vi "Plot_lift_off.vi"() -> ()   [LabVIEW 2018]
panel:
  in  "Raw/Pro":bool
  in  "Backdata":bool=TRUE caption="Scan"
  in  "Exit":bool
  in  "2D Array In":dbl[][](array[numeric])
  in  "Open":bool
  out "Hall sensors signal lf":dbl[][](graph)
  in  "Filter lf":bool=TRUE caption="Scan"
  in  "View Mode":bool caption="Scan"
  in  "Low cutoff freq: fl":dbl
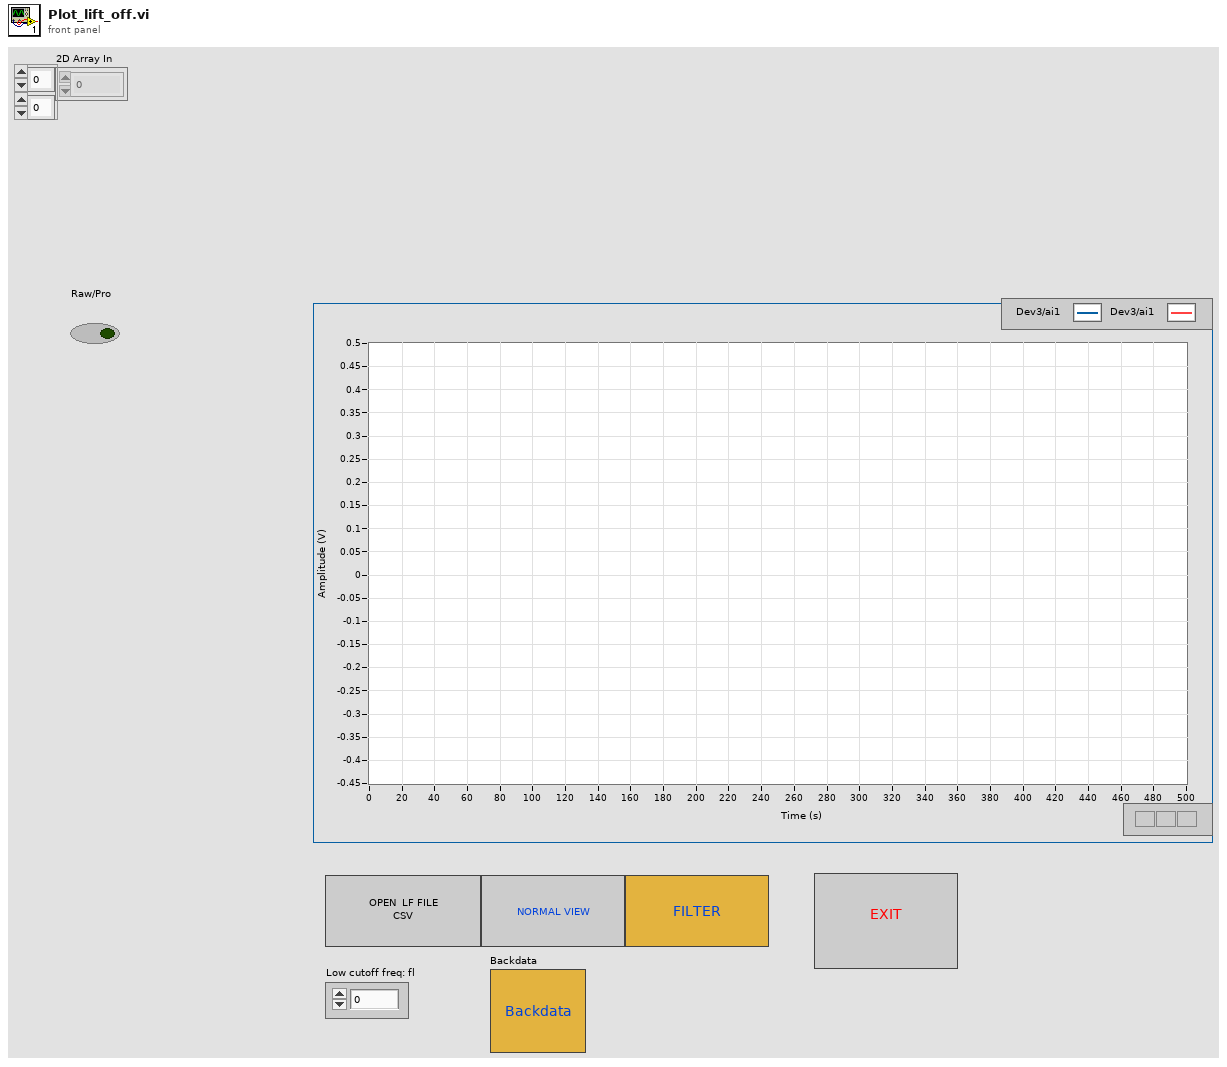
[diagram p1: front panel]
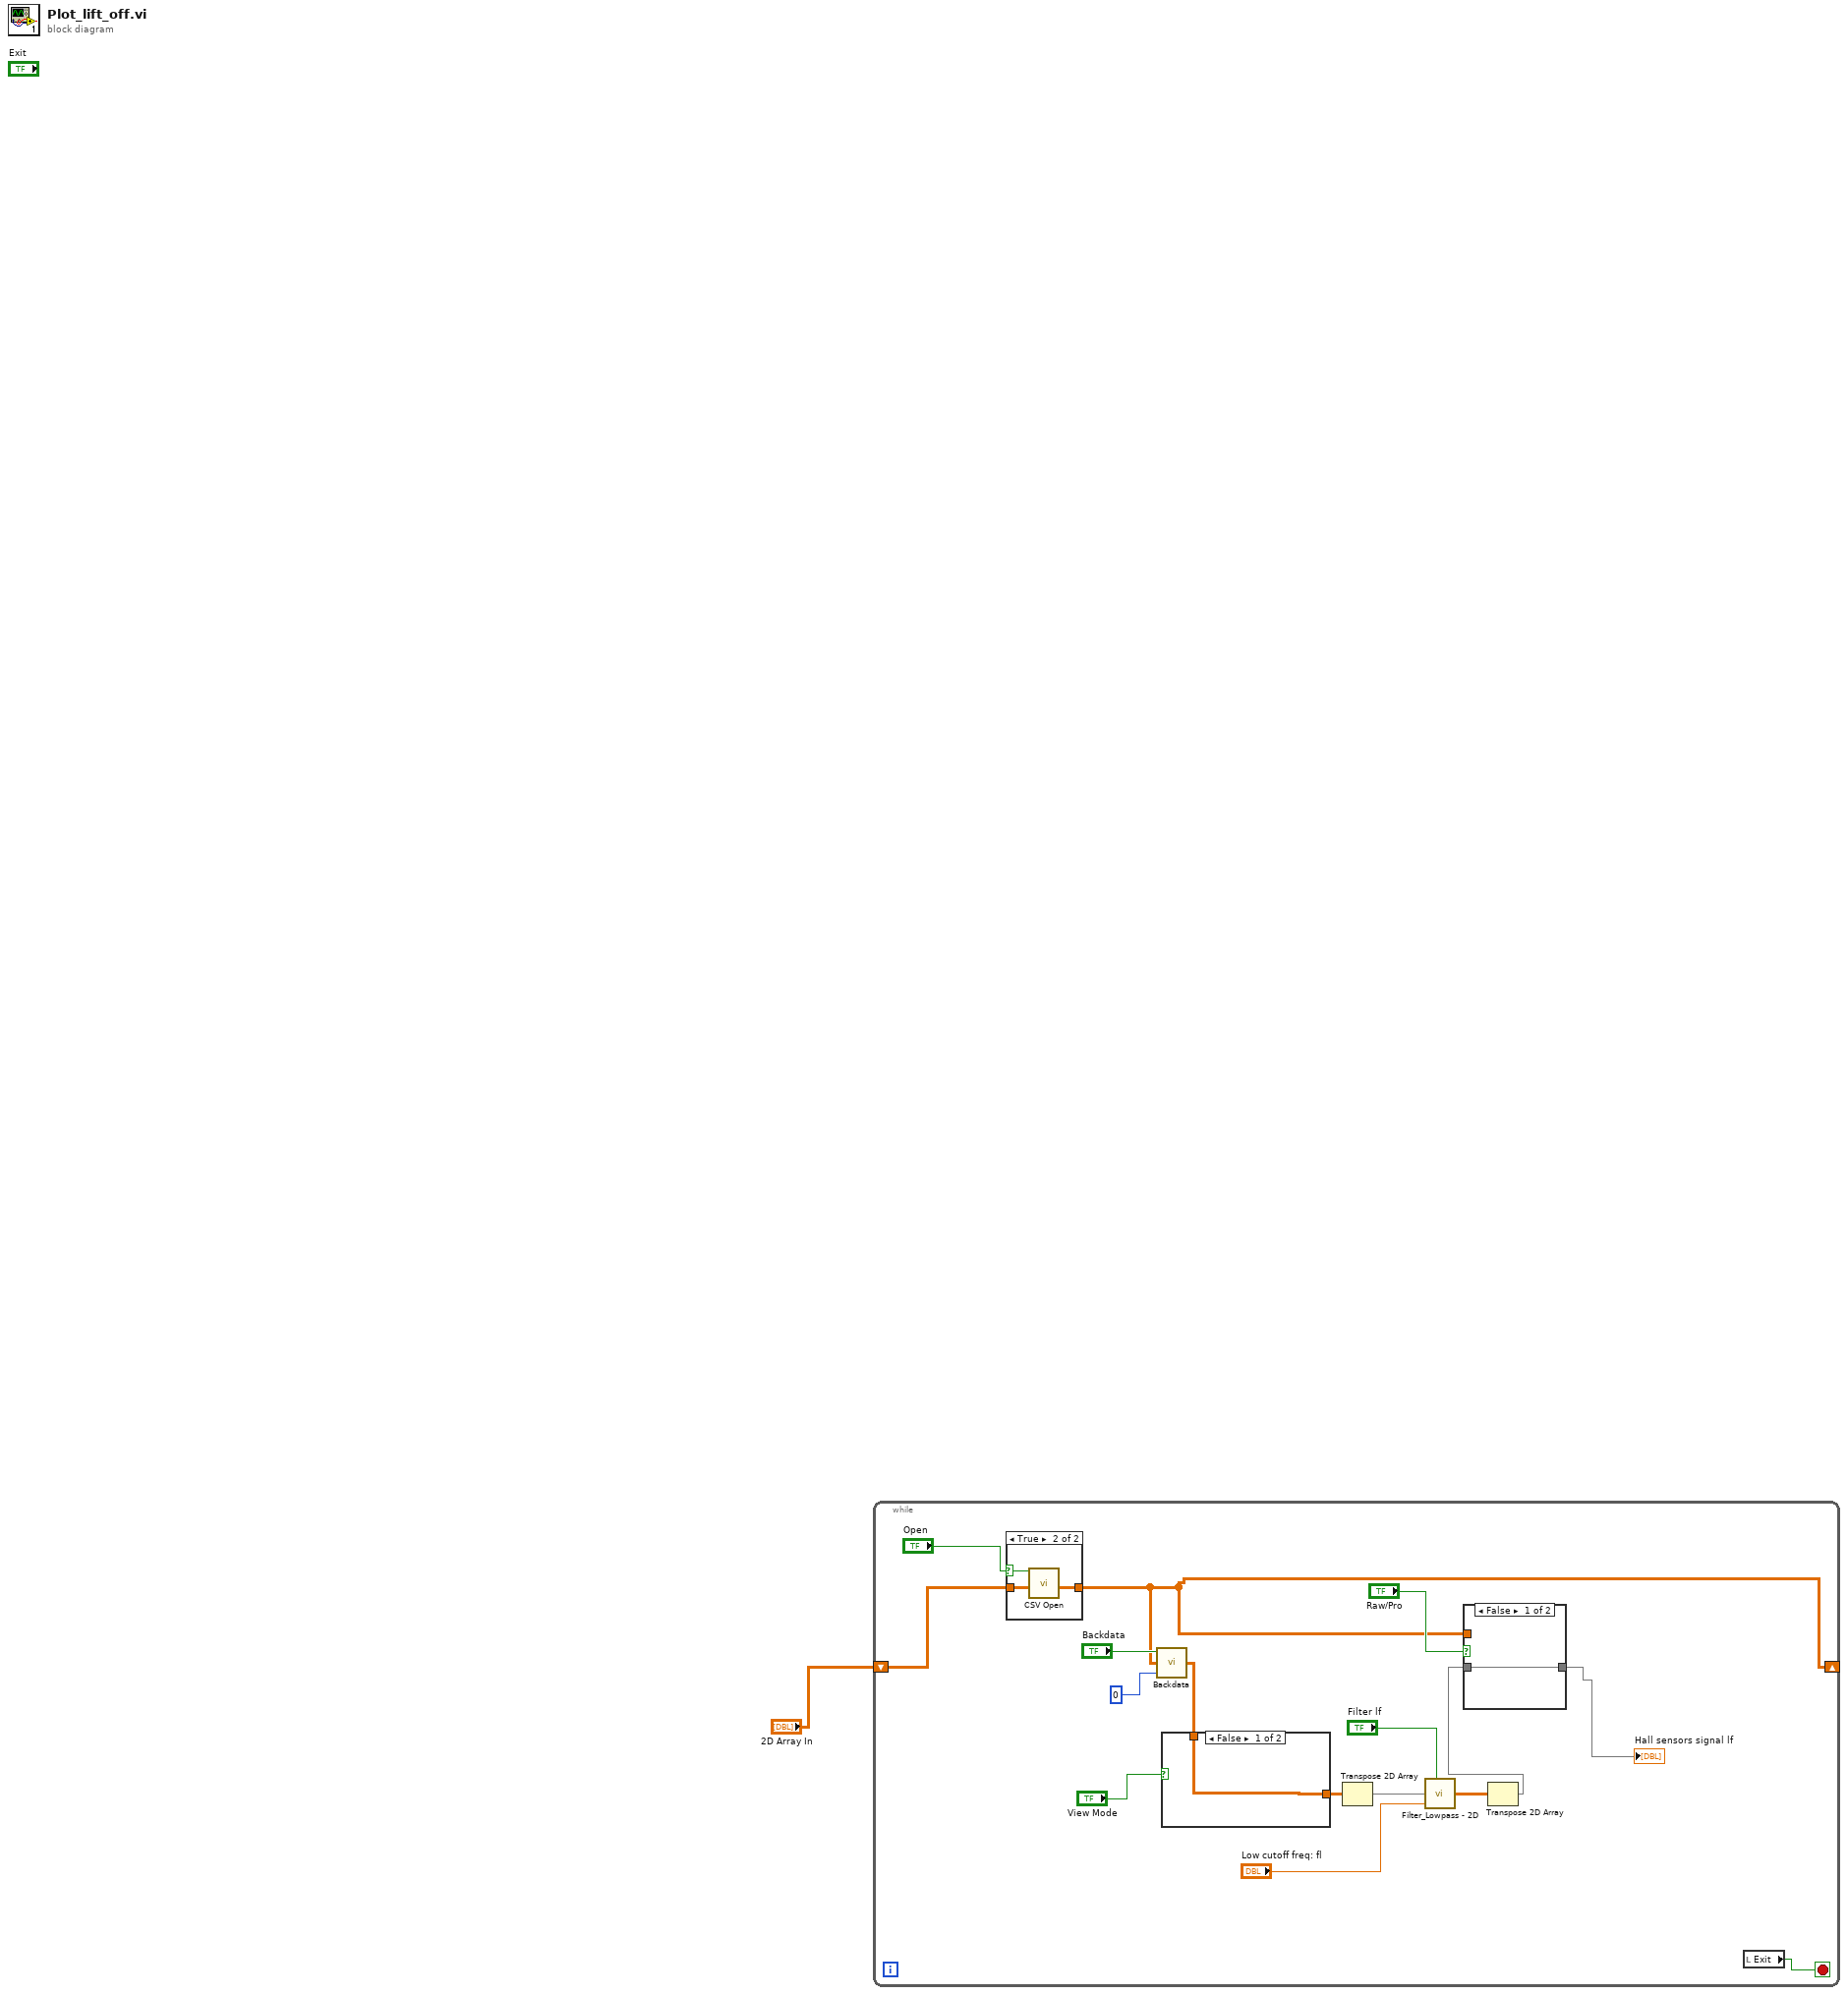
[diagram p0: block diagram]
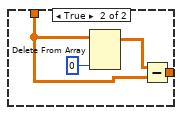
[diagram p4: hidden frame]
diagram:
  n1 = while {
    shift-right: [w2] -> _
    shift-left: "2D Array In" -> [w16]
    stop <- w17 stop-if-true
    n2 = case shown="True" "Open" {
      selector: "Open" -> [_ w21]
      tunnel: w16 -> [w20 w23]
      tunnel: [w20 w22] -> w2
      frame False {
      }
      frame True {
        n3 = call "CSV Open.vi"("2D Array In"=w23, "Open"=w21) -> ("2D Array Out"=w22:dbl[][])  [unwired: 9 in]
      }
    }
    n4 = call "Backdata.vi"("Backindex"=0, "Array in"=w2, "Backdata"="Backdata") -> ("Array out"=w9:dbl[][])
    n5 = case shown="False" "View Mode" {
      tunnel: [w24 w26] -> w15
      tunnel: w9 -> [w24 w25]
      frame False {
      }
      frame True {
        n6 = Delete From Array(array=w25, index (col)=0 ("disabled index (col)")) -> (array with subset deleted=w27:dbl[][])  [unwired: 2 in, 1 out]
        n7 = Subtract(x=w27, y=w25) -> (x-y=w26:dbl[][])
      }
    }
    n8 = Transpose 2D Array(2D array=w15) -> (transposed array=w12:dbl[][])
    n9 = call "Filter_Lowpass - 2D.vi"("Filter"="Filter lf", "Input 2D"=w12, "low cutoff freq: fl"="Low cutoff freq: fl") -> ("Output"=w14:dbl[][])  [unwired: 6 in]
    n10 = Transpose 2D Array(2D array=w14) -> (transposed array=w4:dbl[][])
    n11 = case shown="False" "Raw/Pro" {
      tunnel: w2 -> [_ w19]
      tunnel: [w18 w19] -> w3
      tunnel: w4 -> [w18 _]
      frame False {
      }
      frame True {
      }
    }
    "Hall sensors signal lf" <- w3
    n12 = local read "Exit"() -> (w17:bool)
  }
